vi "_Read Spectrum File.vi"(6 "advisory dialog? (display:T)":bool=TRUE, 8 "Scan#":i32=1, 9 "start path  (Not A Path)":path=path "") -> (0 "error":bool, 1 "TIC":u32, 3 "new file path":path, 4 "error out":errorcluster, 5 "Scan# out":u32=1)   [LabVIEW 2012]
uses:
  Type/_File Command.ctl
  Configuration/_Global Configuration.vi
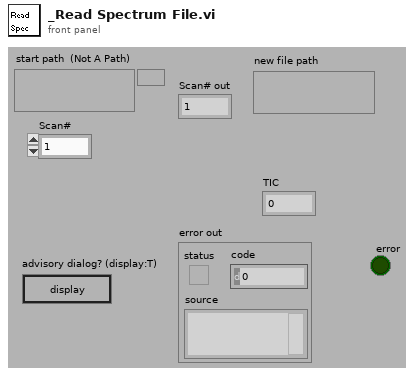
[diagram p1: front panel]
types:
  T1 = typedef "_File Command.ctl" = enum16{"No Command", "Open", "Open Read", "Write", "Get Spectrum", "Close"}
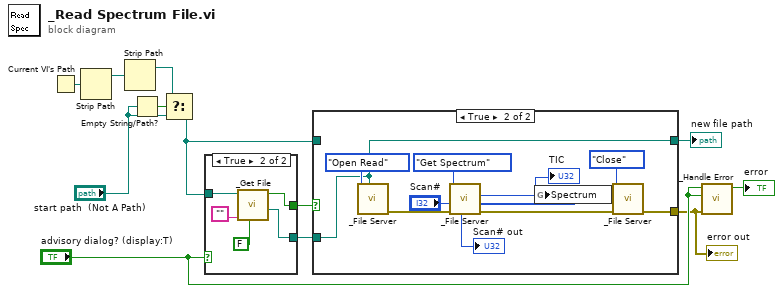
[diagram p0: block diagram]
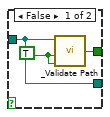
[diagram p3: hidden frame]
diagram:
  n1 = Current VI's Path() -> (path=w10:path)
  n2 = Strip Path(path=w10) -> (stripped path=w9:path)  [unwired: 1 out]
  n3 = Strip Path(path=w9) -> (stripped path=w8:path)  [unwired: 1 out]
  n4 = Empty String/Path?(string/path="start path  (Not A Path)") -> (empty?=w12:bool)
  n5 = Select(t=w8, s=w12, f="start path  (Not A Path)") -> (s? t:f=w4:path)
  n6 = case shown="True" "advisory dialog? (display:T)" {
    tunnel: [w15 w17] -> w3
    tunnel: w4 -> [w15 w20]
    tunnel: [w13 w16] -> w5
    frame False {
      w14 = TRUE
      n7 = call "_Validate Path.vi"("Check Type (F)"=w14, "Check Exist (F)"=w14, "path"=w15) -> ("Valid"=w13:bool)  [unwired: 1 in]
    }
    frame True {
      n8 = call "_Get File.vi"("For Write (T)"=FALSE, "default name"="", "Start Path"=w20) -> ("Seleted File"=w17:path, "Succeeded"=w16:bool)  [unwired: 3 in, 2 out]
    }
  }
  n9 = case shown="True" w5 {
    tunnel: w4 -> [w21 _]
    tunnel: w3 -> [_ w23]
    tunnel: [w21 w23] -> w2
    tunnel: [_ w27] -> w1
    frame False {
    }
    frame True {
      n10 = call "_File Server.vi"("file path"=w23, "File Command"=_File_Command."Open Read") -> ("error out"=w30:errorcluster)  [unwired: 5 in, 4 out]
      n11 = call "_File Server.vi"("error in (no error)"=w30, "Scan#"="Scan#", "File Command"=_File_Command."Get Spectrum") -> ("error out"=w28:errorcluster, "Spectrum Out"=w25:u32[], "TIC"=→"TIC":u32, "Scan# out"=→"Scan# out":i32)  [unwired: 4 in, 1 out]
      n12 = global write "_Global Configuration.vi" "Spectrum"(w25) -> ()
      n13 = call "_File Server.vi"("error in (no error)"=w28, "File Command"=_File_Command."Close") -> ("error out"=w27:errorcluster)  [unwired: 5 in, 4 out]
    }
  }
  "new file path" <- w2
  "error out" <- w1
  n14 = call "_Handle Error.vi"("error in (no error)"=w1, "Display Warning (T)"="advisory dialog? (display:T)", "Display Error (T)"="advisory dialog? (display:T)") -> ("error?"=→"error":bool)  [unwired: 4 out]
